vi "run.property_value_at.vi"(8 "error in":errorcluster, 11 "Run in":refnum<class "Run.lvclass">) -> (0 "error out":errorcluster, 3 "Run out":refnum<class "Run.lvclass">)   [LabVIEW 2020, in "Run.lvclass"]
doc: "Returns the value of the property at the given position in the run's property list."
uses:
  Run.lvclass
  Run.lvclass/Run.ctl
  client.lvlib
panel:
  out "out_needed out":u32
  out "property value":string
  in  "index":i32
  in  "buf":string
  in  "cap":u32
  in  "out_needed":u32
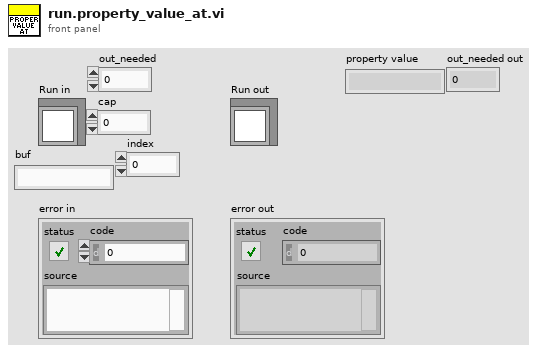
[diagram p1: front panel]
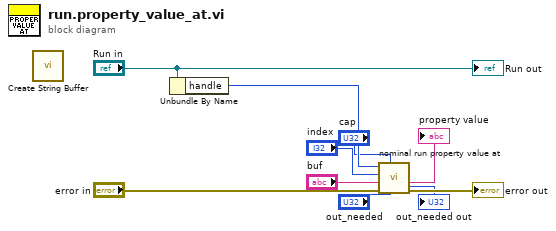
[diagram p0: block diagram]
diagram:
  n1 = call "Create String Buffer.vi"() -> ()  [unwired: 9 in, 3 out]
  n2 = Unbundle By Name("Run in") -> ("handle"=w8:i32)
  n3 = call "nominal run property value at.vi"("out_needed"="out_needed", "cap"="cap", "error in (no error)"="error in", "buf"="buf", "index"="index", "run"=w8) -> ("error out"=→"error out":errorcluster, "buf out"=→"property value":string, "out_needed out"=→"out_needed out":u32)  [unwired: 2 in, 1 out]
  "Run out" <- "Run in"
